vi "FlowChart Edit.vi"(10 "Name":string, 11 "Identifier In":string) -> (0 "Identifiers Out":string[](array[string]), 1 "OK？":bool, 2 "Tips":string, 3 "Identifier Out":string)   [LabVIEW 2020]
uses:
  <vilib>/Utility/miscctls.llb/LVRowAndColumnUnsignedTypeDef.ctl
panel:
  in  "Serrch Info":string
  in  "Search":bool
  in  "Data List":i32[](listbox)
  in  "OK":bool
  in  "Cancel":bool
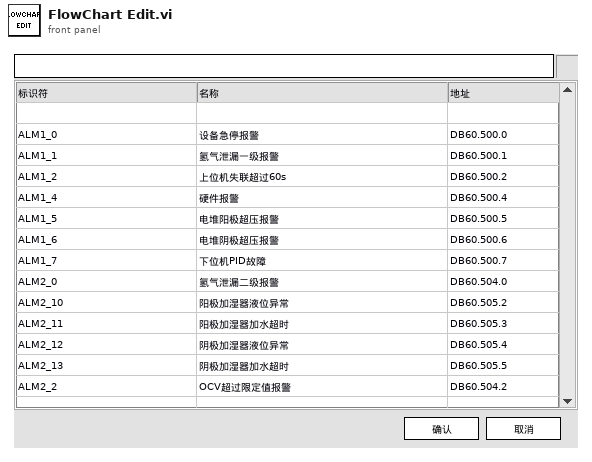
[diagram p1: front panel]
types:
  T1 = typedef "LVRowAndColumnUnsignedTypeDef.ctl" = cluster{"Row":u32, "Column":u32}
  T2 = enum32{"Invalid", "Default", "Floating", "Floating/Auto-Hide", "Modal"}
  T3 = typedef "SDQ Data Type.ctl" = cluster{"CAN Length":string, "CAN Name":string, "CAN ID":string, "CAN Type":string, "Test Item":string, "Byte Order":string, "Instruction":string, "Control Type":string, "Group":string, "Offset":dbl, "Coefficient":dbl, "Write Enable":bool, "Lable Type":string, "Key?":string, "Set Value":string, "Upper":dbl, "Lower":dbl, "Unit":string, "Formula":string, "Test Item Type":string, "Length":i32, "Address":string, "Name":string, "Identifier":string, "Data Type":string, "Enumerate?":string, "Enumerate List":string, "Data":string, "Source":string}
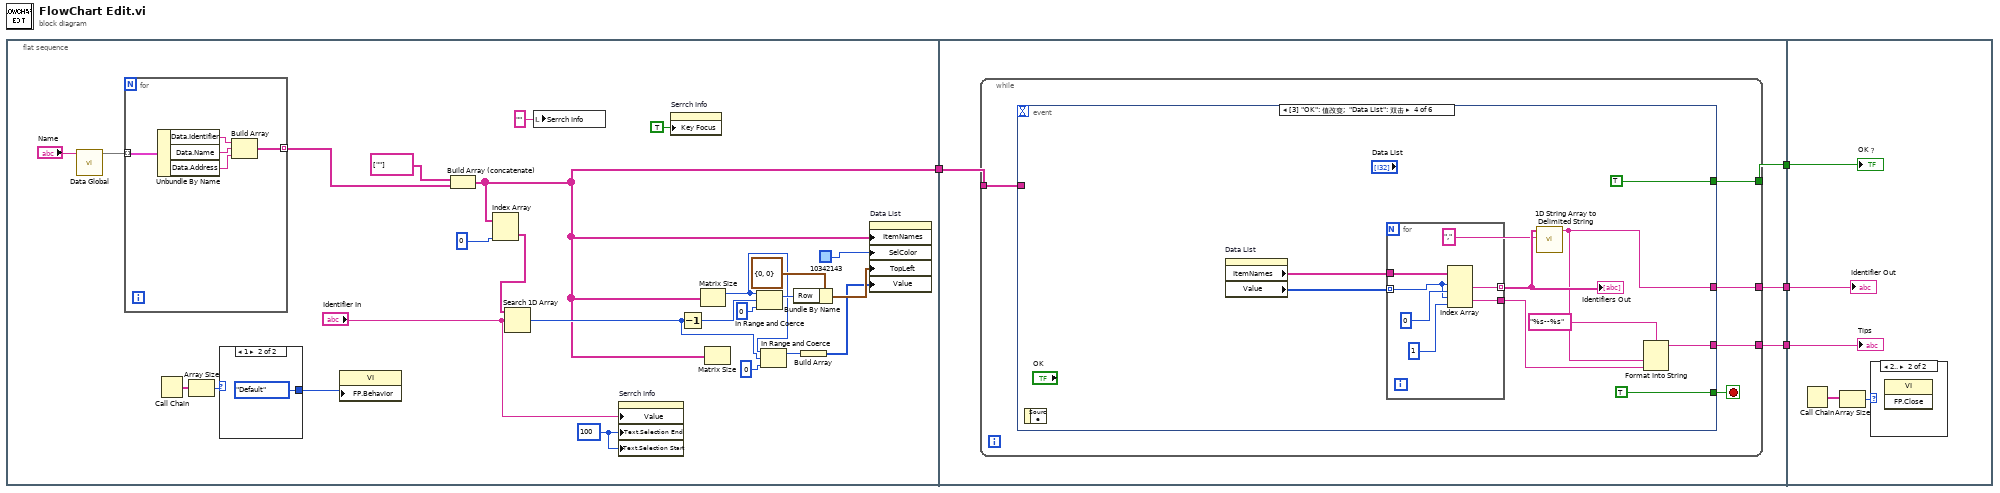
[diagram p0: block diagram]
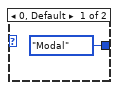
[diagram p2: hidden frame]
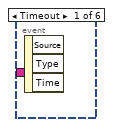
[diagram p3: hidden frame]
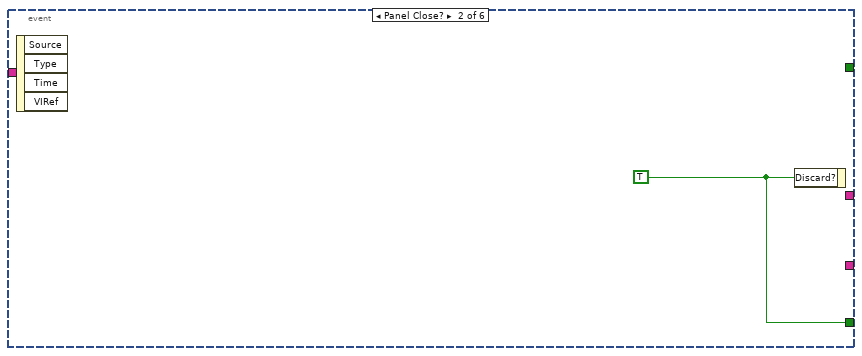
[diagram p4: hidden frame]
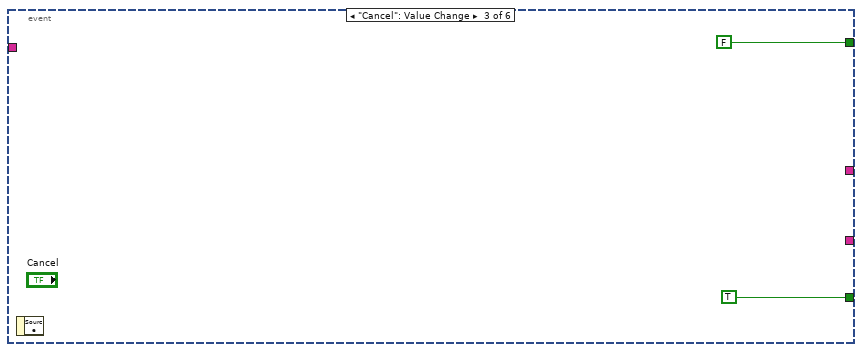
[diagram p5: hidden frame]
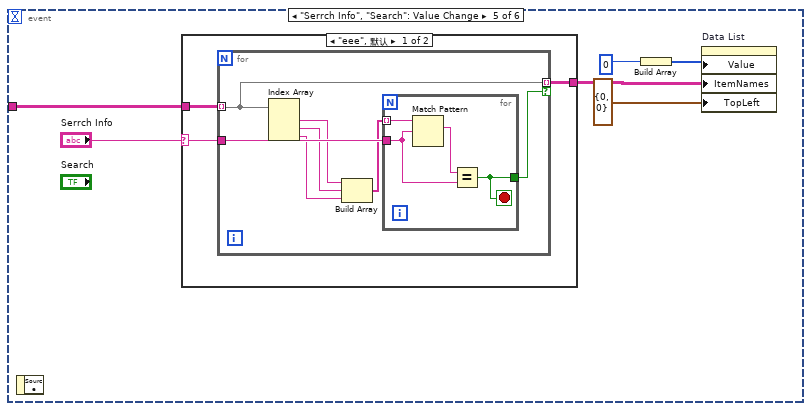
[diagram p6: hidden frame]
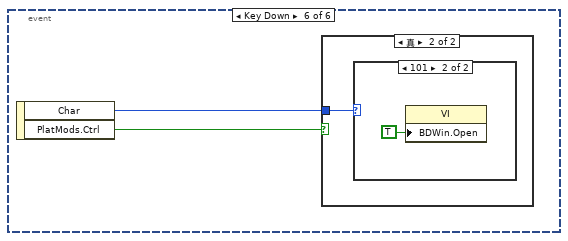
[diagram p8: hidden frame]
diagram:
  n1 = flat-sequence {
    tunnel: [w9] -> w1
    tunnel: [w40] -> w4
    tunnel: [w39] -> w3
    tunnel: [w38] -> w2
    tunnel: w1 -> [w37]
    tunnel: w4 -> [w94]
    tunnel: w3 -> [w93]
    tunnel: w2 -> [w90]
    frame #0 {
      w20 = u32 100 ("文本.选择区域:末尾")
      n2 = call "Data Global.vi"("Name"="Name") -> ("Data Out"=w6:map{string, T3})  [unwired: 7 in, 3 out]
      n3 = for {
        tunnel: w6 -> [w36] mode=indexing
        tunnel: [w33] -> w11 mode=indexing
        n4 = Unbundle By Name(w36) -> ("Data.Identifier"=w32:string, "Data.Name"=w35:string, "Data.Address"=w34:string)
        n5 = Build Array(w32, w35, w34) -> (w33:string[])
      }
      n6 = Call Chain() -> (call chain=w14:string[])
      n7 = Array Size(array=w14) -> (size(s)=w13:i32)
      n8 = case shown="1" w13 {
        tunnel: [T2."Modal" ("前面板窗口:动作") T2."Default" ("前面板窗口:动作")] -> w12
        frame 0, Default {
        }
        frame 1 {
        }
      }
      n9 = property class="VI"("FP.Behavior"=w12) -> ()  [unwired: 2 in, 2 out]
      n10 = Build Array (concatenate)(string[] [""] ("Serrch Info"), w11) -> (w9:string[][])
      n11 = Index Array(array=w9, index (col)=0 ("索引 (行)")) -> (element=w8:string[])  [unwired: 1 in]
      n12 = Search 1D Array(1D array=w8, element="Identifier In") -> (index of element=w17:i32)  [unwired: 1 in]
      n13 = local write "Serrch Info"("" ("Serrch Info")) -> ()
      n14 = property on="Serrch Info" class="Str"("Value"="Identifier In", "Text.Selection End"=w20, "Text.Selection Start"=w20) -> ()  [unwired: 2 in, 2 out]
      n15 = property on="Serrch Info" class="Str"("Key Focus"=TRUE ("键选中")) -> ()  [unwired: 2 in, 2 out]
      n16 = Decrement(x=w17) -> (x-1=w25:i32)
      n17 = Matrix Size(0:w9) -> (1:w18:i32)  [unwired: 1 out]
      n18 = Matrix Size(0:w9) -> ()  [unwired: 2 out]
      n19 = In Range and Coerce(upper limit=w18, x=w25, lower limit=0 ("x-1")) -> (coerced(x)=w24:i32)  [unwired: 1 out]
      n20 = In Range and Coerce(upper limit=w18, x=w17, lower limit=0 ("x-1")) -> (coerced(x)=w16:i32)  [unwired: 1 out]
      n21 = Bundle By Name(cluster=T1 {"Row"=0, "Column"=0} ("左上可见单元格"), "Row"=w24) -> (w27:T1)
      n22 = Build Array(w16) -> (w15:i32[])
      n23 = property on="Data List" class="MCListbox (严格)"("ItemNames"=w9, "SelColor"=u32 10342143 ("选择颜色"), "TopLeft"=w27, "Value"=w15) -> ()  [unwired: 2 in, 2 out]
    }
    frame #1 {
      n24 = while {
        tunnel: [w44] -> w40
        tunnel: [w43] -> w39
        tunnel: [w42] -> w38
        tunnel: w37 -> [w41]
        stop <- w45 stop-if-true
        n25 = event shown="[3] \"OK\": 值改变;  \"Data List\": 双击" {
          selector: _ -> [_ _ _ _ _ _]
          dyn-events: _ -> [_ _ _ _ _ _]
          timeout: _ -> [_ _ _ _ _ _]
          tunnel: [_ w46 TRUE ("放弃？") TRUE ("放弃？") _ _] -> w45
          tunnel: [_ _ FALSE TRUE _ _] -> w44
          tunnel: [_ _ _ w49 _ _] -> w43
          tunnel: [_ _ _ w52 _ _] -> w42
          tunnel: w41 -> [_ _ _ _ w70 _]
          event Timeout {
            n26 = event-data() -> ()  [unwired: 1 in, 3 out]
          }
          event Panel Close? {
            w46 = TRUE ("放弃？")
            n27 = event-data() -> ()  [unwired: 1 in, 4 out]
            n28 = event-data("Discard?"=w46) -> ()  [unwired: 1 in, 1 out]
          }
          event "Cancel": Value Change {
            n29 = event-data() -> ()  [unwired: 1 in, 1 out]
          }
          event "OK": Value Change; "Data List": Double Click {
            n30 = event-data() -> ()  [unwired: 1 in, 1 out]
            n31 = property on="Data List" class="MCListbox (严格)"() -> ("ItemNames"=w56:string[][], "Value"=w55:i32[])  [unwired: 2 in, 2 out]
            n32 = for {
              tunnel: w56 -> [w64]
              tunnel: w55 -> [w62] mode=indexing
              tunnel: [w60] -> w51 mode=indexing
              tunnel: [w59] -> w53
              n33 = Index Array(array=w64, index (row) #1=w62, index (col) #1=0 ("禁用的索引 (列)"), index (row) #2=w62, index (col) #2=1 ("禁用的索引 (列)")) -> (element #1=w60:string, element #2=w59:string)
            }
            "Identifiers Out" <- w51
            n34 = call <vilib>:"1D String Array to Delimited String.vi"("delimiter"=",", "string array"=w51) -> ("delimited string"=w49:string)  [unwired: 9 in]
            n35 = Format Into String(format string="%s--%s" ("格式字符串"), w49, w53) -> (resulting string=w52:string)  [unwired: 2 in, 1 out]
          }
          event "Serrch Info", "Search": Value Change {
            n36 = event-data() -> ()  [unwired: 1 in, 1 out]
            n37 = case shown="\"eee\", 默认" "Serrch Info" {
              selector: "Serrch Info" -> [w72 _]
              tunnel: w70 -> [w73 w85]
              tunnel: [w71 w85] -> w68
              frame "eee", Default {
                n38 = for {
                  tunnel: w73 -> [w79] mode=indexing
                  tunnel: w72 -> [w80]
                  tunnel: [w79] -> w71 mode=indexing if=w78
                  n39 = Index Array(array=w79) -> (element #1=w77:string, element #2=w76:string, element #3=w75:string)  [unwired: 3 in]
                  n40 = Build Array(w77, w76, w75) -> (w74:string[])
                  n41 = for {
                    tunnel: w80 -> [w83]
                    tunnel: [w81] -> w78
                    tunnel: w74 -> [w82] mode=indexing
                    stop <- w81 stop-if-true
                    n42 = Match Pattern(string=w82, regular expression=w83) -> (match substring=w84:string)  [unwired: 1 in, 3 out]
                    n43 = Equal?(x=w84, y=w83) -> (x = y?=w81:bool)
                  }
                }
              }
              frame "" {
              }
            }
            n44 = Build Array(0 ("Data List")) -> (w65:i32[])
            n45 = property on="Data List" class="MCListbox (严格)"("Value"=w65, "ItemNames"=w68, "TopLeft"=T1 {"Row"=0, "Column"=0} ("左上可见单元格")) -> ()  [unwired: 2 in, 2 out]
          }
          event Key Down {
            n46 = event-data() -> ("Char"=w86:i16, "PlatMods.Ctrl"=w87:bool)  [unwired: 1 in]
            n47 = case shown="真" w87 {
              tunnel: w86 -> [_ w88]
              frame False {
              }
              frame True {
                n48 = case shown="101" w88 {
                  frame 0, Default {
                  }
                  frame 101 {
                    n49 = property class="VI"("BDWin.Open"=TRUE ("程序框图窗口:打开")) -> ()  [unwired: 2 in, 2 out]
                  }
                }
              }
            }
          }
        }
      }
    }
    frame #2 {
      n50 = Call Chain() -> (call chain=w92:string[])
      n51 = Array Size(array=w92) -> (size(s)=w91:i32)
      n52 = case shown="2.." w91 {
        frame 0, Default {
        }
        frame 2.. {
          n53 = invoke class="VI" method="FP.Close"() -> ()  [unwired: 3 in, 3 out]
        }
      }
      "OK？" <- w94
      "Identifier Out" <- w93
      "Tips" <- w90
    }
  }
